vi "CoerceWL.vi"(6 "calType":enum16{"INTERNAL_CAL", "FULL_CAL"}(ring), 8 "Parameter Type":enum16{"Calibration", "Scan"}(ring), 9 "wlType":enum16{"Center WL", "Start WL"}(ring), 10 "Wavelength Range (nm)":refnum<vi>, 11 "Start/Center Wavelength (nm)":dbl=1550.0 format="%.8f") -> (0 "end WL (nm)":dbl format="%.8f", 1 "start WL (nm)":dbl format="%.8f", 2 "Scan Range String":string, 3 "Center WL -- Out":dbl format="%.8f")   [LabVIEW 2024]
uses:
  OVA32.dll
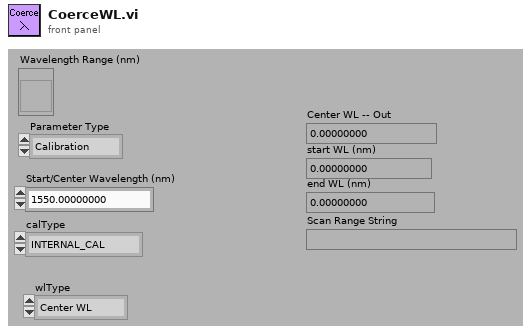
[diagram p1: front panel]
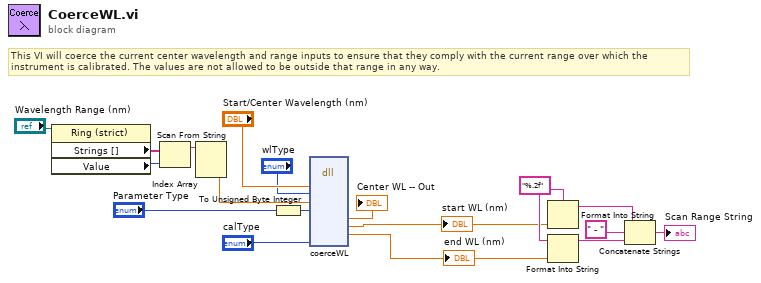
[diagram p0: block diagram]
diagram:
  w14 = "%.2f" ("Format String")
  # "This VI will coerce the current center wavelength and range inputs to ensure that they comply with the current range over which the\ninstrument is calibrated. The values are not allowed to be outside that range in any way."
  n1 = property class="Ring (strict)"(reference="Wavelength Range (nm)") -> ("Strings []"=w16:string[], "Value"=w18:u16)  [unwired: 1 in, 2 out]
  n2 = Index Array(array=w16, index=w18) -> (element=w17:string)
  n3 = Scan From String(input string=w17) -> (output 1=w5:dbl)  [unwired: 4 in, 3 out]
  n4 = To Unsigned Byte Integer(number="Parameter Type") -> (unsigned 8bit integer=w7:u8)
  n5 = dll-call lib="OVA32.dll" fn="coerceWL"("wavelength"="Start/Center Wavelength (nm)", "wlType"="wlType", "reqRange"=w5, "scanType"=w7, "calType"="calType") -> ("centerWl"=→"Center WL -- Out":dbl, "startWL"=w1:dbl, "endWL"=w2:dbl)  [unwired: 12 in, 2 out]
  "start WL (nm)" <- w1
  "end WL (nm)" <- w2
  n6 = Format Into String(format string=w14, w1) -> (resulting string=w13:string)  [unwired: 2 in, 1 out]
  n7 = Format Into String(format string=w14, w2) -> (resulting string=w12:string)  [unwired: 2 in, 1 out]
  n8 = Concatenate Strings(w13, " - ", w12) -> (→"Scan Range String":string)
